vi "Create Child Element.vi"(8 "error in (no error)":errorcluster, 9 "Value (\"\")":string, 10 "Name":string="testsuite", 11 "Element in":refnum<k20>) -> (0 "error out":errorcluster, 2 "Child Element":refnum<k20>, 3 "Element out":refnum<k20>)   [LabVIEW 2013, in "XML.lvlib"]
doc: "Creates a new child element with the specified name and value under the current element and returns the created element. The caller is responsible for cleaning up references."
uses:
  XML.lvlib
  <vilib>/xml/Close Reference(Node).vi
  <resource>/objmgr/DOMUserDefRef.rc
  <vilib>/xml/NI_XML.lvlib
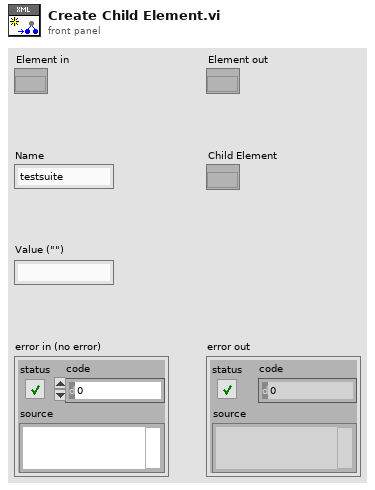
[diagram p1: front panel]
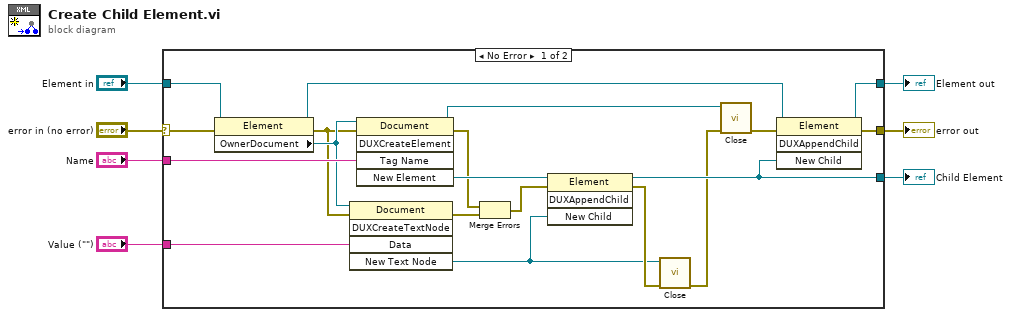
[diagram p0: block diagram]
diagram:
  n1 = case shown="No Error" "error in (no error)" {
    selector: "error in (no error)" -> [w23 w28]
    tunnel: [w11 _] -> w7
    tunnel: "Element in" -> [w22 w27]
    tunnel: [w26 w27] -> w5
    tunnel: "Name" -> [w25 _]
    tunnel: [w24 w28] -> w3
    tunnel: "Value (\"\")" -> [w20 _]
    frame No Error {
      n2 = property class="Element"(reference=w22, error in=w23) -> (reference out=w21:refnum<k20>, error out=w17:errorcluster, "OwnerDocument"=w18:refnum<k20>)
      n3 = invoke class="Document" method="DUXCreateTextNode"(reference=w18, error in=w17, "Data"=w20) -> (error out=w15:errorcluster, "New Text Node"=w12:refnum<k20>)  [unwired: 2 in, 3 out]
      n4 = invoke class="Document" method="DUXCreateElement"(reference=w18, error in=w17, "Tag Name"=w25) -> (reference out=w8:refnum<k20>, error out=w16:errorcluster, "New Element"=w19:refnum<k20>)  [unwired: 2 in, 2 out]
      n5 = Merge Errors(w16, w15) -> (w14:errorcluster)
      n6 = invoke class="Element" method="DUXAppendChild"(reference=w19, error in=w14, "New Child"=w12) -> (reference out=w11:refnum<k20>, error out=w13:errorcluster)  [unwired: 1 in, 2 out]
      n7 = call-poly <vilib>:"Close.vi"("error in (no error)"=w13, "node"=w12) -> ("error out"=w9:errorcluster)  [unwired: 7 in]
      n8 = call-poly <vilib>:"Close.vi"("error in (no error)"=w9, "node"=w8) -> ("error out"=w10:errorcluster)  [unwired: 7 in]
      n9 = invoke class="Element" method="DUXAppendChild"(reference=w21, error in=w10, "New Child"=w11) -> (reference out=w26:refnum<k20>, error out=w24:errorcluster)  [unwired: 1 in, 2 out]
    }
    frame Error {
    }
  }
  "Element out" <- w5
  "Child Element" <- w7
  "error out" <- w3
